vi "AMB_TCP_Find_Slaves.vi"(0 "ObjHandle In":u32, 1 "error in":errorcluster {"code" format="%.0x"}) -> (2 "ObjHandle Out":u32, 3 "NumSlaves out":u8, 4 "Node Array out":cluster{"Address":i8, "Serial Number":i8[]}[](array[cluster]) {"Serial Number" format="%.0x"}, 5 "error out":errorcluster {"code" format="%.0x"})   [LabVIEW 2017]
doc: "This VI finds all of the AMB slaves currently active on the CAN network.\nYou should have already setup the AMB with the AMB Setup VI."
uses:
  AMB_Global.gbl.vi
panel:
  in  "CAN ID in":u32 format="%.0x"
  in  "TCP Connection ID":refnum<k5>
  # "ALMA Monitor and Control Bus\nFind Slave Nodes"
  # "Node Address"
  # "Serial Number"
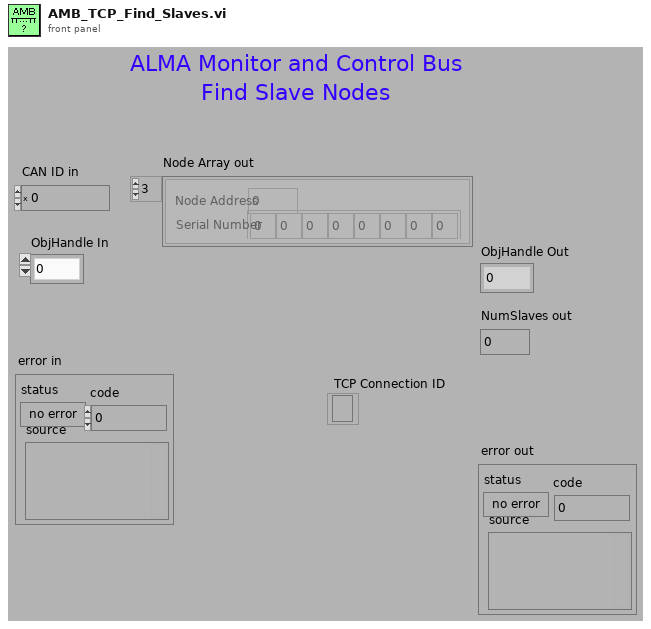
[diagram p1: front panel]
types:
  T1 = enum16{"Standard", "Buffered", "CRLF", "Immediate"}
  T2 = cluster{"status":bool, "code":i32, "concatenated string":string}
  T3 = cluster{"status":bool, "code":i32, "String To Add":string}
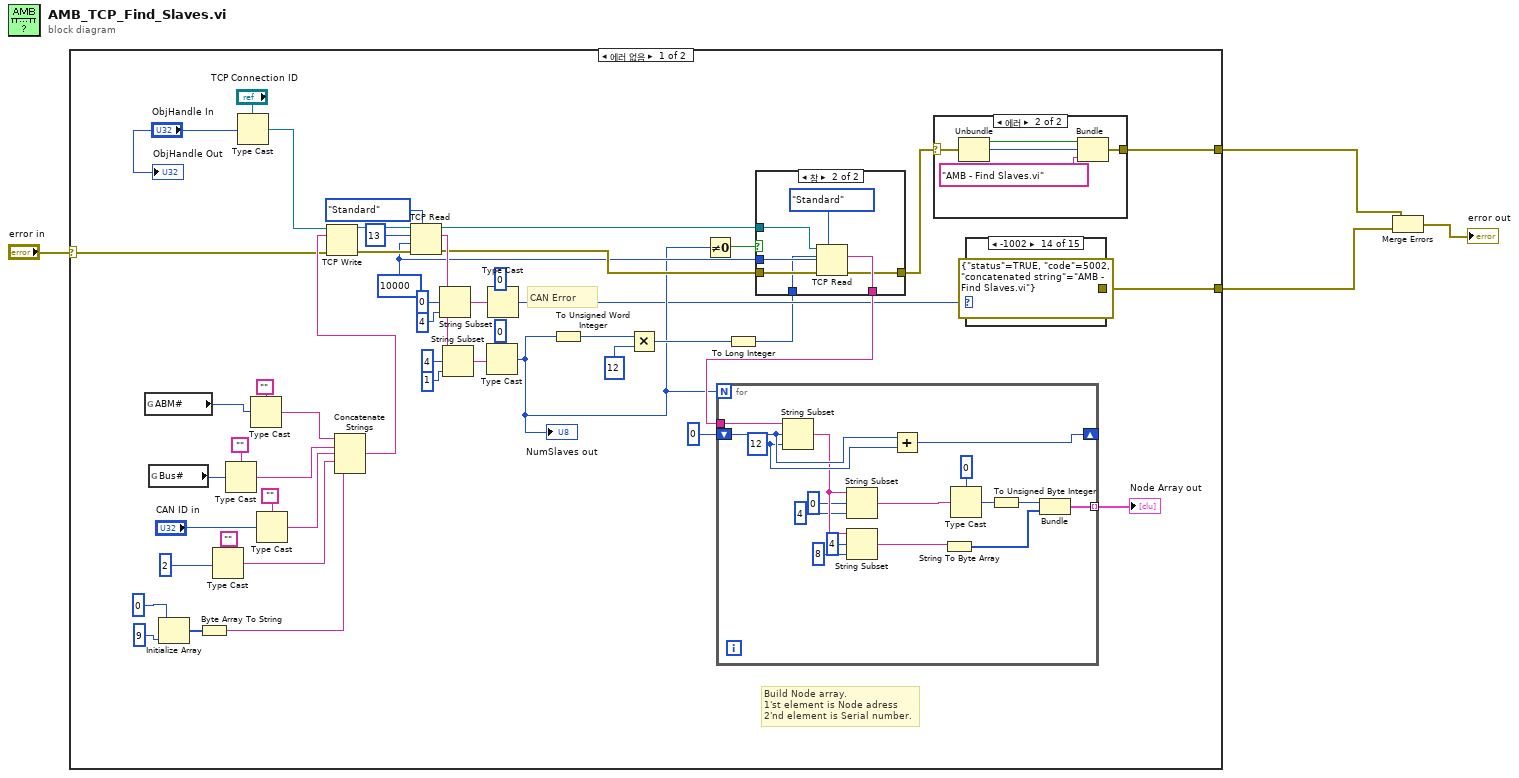
[diagram p0: block diagram]
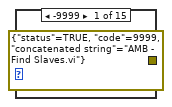
[diagram p3: hidden frame]
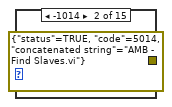
[diagram p4: hidden frame]
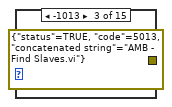
[diagram p5: hidden frame]
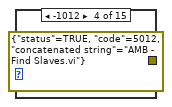
[diagram p6: hidden frame]
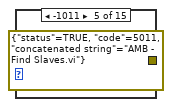
[diagram p7: hidden frame]
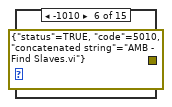
[diagram p8: hidden frame]
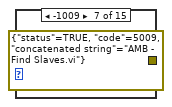
[diagram p9: hidden frame]
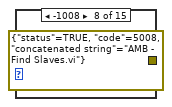
[diagram p10: hidden frame]
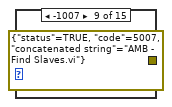
[diagram p11: hidden frame]
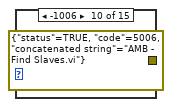
[diagram p12: hidden frame]
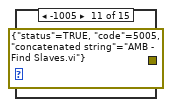
[diagram p13: hidden frame]
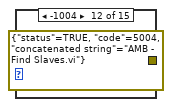
[diagram p14: hidden frame]
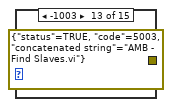
[diagram p15: hidden frame]
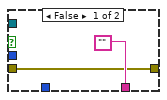
[diagram p17: hidden frame]
diagram:
  n1 = case shown="에러 없음" "error in" {
    selector: "error in" -> [w11 w100]
    tunnel: [w9 w100] -> w2
    tunnel: [w8 _] -> w1
    frame No Error {
      w17 = 10000 ("timeout ms (25000)")
      # "CAN Error"
      # "Build Node array.\n1'st element is Node adress\n2'nd element is Serial number."
      n2 = global read "AMB_Global.gbl.vi" "ABM#"() -> (w41:i16)
      n3 = global read "AMB_Global.gbl.vi" "Bus#"() -> (w40:u16)
      n4 = Initialize Array(0, 9) -> (w37:i32[])
      n5 = Byte Array To String(unsigned byte array=w37) -> (string=w21:string)
      n6 = Type Cast(type="", x=u8 2) -> (*(type *) &x=w20:string)
      n7 = Type Cast(type="", x=w40) -> (*(type *) &x=w35:string)
      n8 = Type Cast(type="TCP Connection ID", x="ObjHandle In") -> (*(type *) &x=w46:refnum<k5>)
      n9 = Type Cast(type="", x=w41) -> (*(type *) &x=w36:string)
      n10 = Type Cast(type="", x="CAN ID in") -> (*(type *) &x=w34:string)
      n11 = Concatenate Strings(w36, w35, w34, w20, w21) -> (w33:string)
      n12 = TCP Write(connection ID=w46, data in=w33, error in (no error)=w11) -> (connection ID out=w54:refnum<k5>, error out=w52:errorcluster)  [unwired: 1 in, 1 out]
      n13 = TCP Read(connection ID=w54, bytes to read=13, error in (no error)=w52, 7:T1."Standard" ("mode (standard)"), 9:w17) -> (connection ID out=w19:refnum<k5>, data out=w24:string, error out=w18:errorcluster)
      n14 = String Subset(string=w24, offset (0)=0, length (rest)=4 ("length (rest)")) -> (substring=w29:string)
      n15 = String Subset(string=w24, offset (0)=4, length (rest)=1 ("length (rest)")) -> (substring=w25:string)
      n16 = Type Cast(type=u8 0, x=w25) -> (*(type *) &x=w13:u8)
      "NumSlaves out" <- w13
      n17 = Type Cast(type=0, x=w29) -> (*(type *) &x=w12:i32)
      n18 = To Unsigned Word Integer(number=w13) -> (unsigned 16bit integer=w5:u16)
      n19 = Multiply(x=w5, y=u16 12) -> (x*y=w16:u16)
      n20 = Not Equal To 0?(x=w13) -> (x != 0?=w14:bool)
      n21 = To Long Integer(number=w16) -> (32bit integer=w6:i32)
      n22 = case shown="참" w14 {
        tunnel: w19 -> [_ w83]
        tunnel: w18 -> [w75 w82]
        tunnel: w17 -> [_ w81]
        tunnel: w6 -> [_ w80]
        tunnel: ["" w79] -> w15
        tunnel: [w75 w77] -> w10
        frame False {
        }
        frame True {
          n23 = TCP Read(connection ID=w83, bytes to read=w80, error in (no error)=w82, 7:T1."Standard" ("mode (standard)"), 9:w81) -> (data out=w79:string, error out=w77:errorcluster)  [unwired: 1 out]
        }
      }
      n24 = for {
        N: w13 -> [_]
        shift-right: [w97] -> _
        shift-left: 0 ("offset (0)") -> [w99]
        tunnel: w15 -> [w96]
        tunnel: [w87] -> w7 mode=indexing
        w98 = 12 ("length (rest)")
        n25 = String Subset(string=w96, offset (0)=w99, length (rest)=w98) -> (substring=w95:string)
        n26 = String Subset(string=w95, offset (0)=0, length (rest)=4 ("length (rest)")) -> (substring=w86:string)
        n27 = String Subset(string=w95, offset (0)=4, length (rest)=8 ("length (rest)")) -> (substring=w85:string)
        n28 = Add(x=w99, y=w98) -> (x+y=w97:i32)
        n29 = String To Byte Array(string=w85) -> (unsigned byte array=w84:u8[])
        n30 = Type Cast(type=u32 0, x=w86) -> (*(type *) &x=w89:u32)
        n31 = To Unsigned Byte Integer(number=w89) -> (unsigned 8bit integer=w88:u8)
        n32 = Bundle(w88, "unsigned byte array"=w84) -> (w87:cluster{u8, "unsigned byte array":u8[]})  [unwired: 1 in]
      }
      "Node Array out" <- w7
      n33 = case shown="에러" w10 {
        selector: w10 -> [w55 w60]
        tunnel: [w55 w57] -> w9
        frame No Error {
        }
        frame Error {
          n34 = Unbundle(w60) -> ("status"=w59:bool, "code"=w58:i32)  [unwired: 1 out]
          n35 = Bundle("status"=w59, "code"=w58, "String To Add"="AMB - Find Slaves.vi") -> (w57:T3)  [unwired: 1 in]
        }
      }
      n36 = case shown="-1002" w12 {
        tunnel: [T2 {"status"=TRUE, "code"=9999, "concatenated string"="AMB - Find Slaves.vi"} ("output cluster") T2 {"status"=TRUE, "code"=5014, "concatenated string"="AMB - Find Slaves.vi"} ("output cluster") T2 {"status"=TRUE, "code"=5013, "concatenated string"="AMB - Find Slaves.vi"} ("output cluster") T2 {"status"=TRUE, "code"=5012, "concatenated string"="AMB - Find Slaves.vi"} ("output cluster") T2 {"status"=TRUE, "code"=5011, "concatenated string"="AMB - Find Slaves.vi"} ("output cluster") T2 {"status"=TRUE, "code"=5010, "concatenated string"="AMB - Find Slaves.vi"} ("output cluster") T2 {"status"=TRUE, "code"=5009, "concatenated string"="AMB - Find Slaves.vi"} ("output cluster") T2 {"status"=TRUE, "code"=5008, "concatenated string"="AMB - Find Slaves.vi"} ("output cluster") T2 {"status"=TRUE, "code"=5007, "concatenated string"="AMB - Find Slaves.vi"} ("output cluster") T2 {"status"=TRUE, "code"=5006, "concatenated string"="AMB - Find Slaves.vi"} ("output cluster") T2 {"status"=TRUE, "code"=5005, "concatenated string"="AMB - Find Slaves.vi"} ("output cluster") T2 {"status"=TRUE, "code"=5004, "concatenated string"="AMB - Find Slaves.vi"} ("output cluster") T2 {"status"=TRUE, "code"=5003, "concatenated string"="AMB - Find Slaves.vi"} ("output cluster") T2 {"status"=TRUE, "code"=5002, "concatenated string"="AMB - Find Slaves.vi"} ("output cluster") _] -> w8
        frame -9999 {
        }
        frame -1014 {
        }
        frame -1013 {
        }
        frame -1012 {
        }
        frame -1011 {
        }
        frame -1010 {
        }
        frame -1009 {
        }
        frame -1008 {
        }
        frame -1007 {
        }
        frame -1006 {
        }
        frame -1005 {
        }
        frame -1004 {
        }
        frame -1003 {
        }
        frame -1002 {
        }
        frame 0, Default {
        }
      }
      "ObjHandle Out" <- "ObjHandle In"
    }
    frame Error {
    }
  }
  n37 = Merge Errors(w2, w1) -> (→"error out":errorcluster)
